vi "Close MeasurementLink Session.vi"(8 "error in":errorcluster, 9 "initialize and close session behavior":T1, 10 "session in":variant, 11 "instrument in":refnum<class "Instrument.lvclass">) -> (0 "error out":errorcluster)   [LabVIEW 2020, in "MeasurementLink niDMM.lvlib" / "Instrument.lvclass"]
uses:
  Instrument.lvclass
  MeasurementLink Measurement Server/Helpers/Error Strings Global Internal.vi
  Instrument.lvclass/Instrument.ctl
  MeasurementLink Instrument/IInstrument/IInstrument.lvclass
  MeasurementLink Instrument/IInstrument/Initialize and Close Session Behavior.ctl
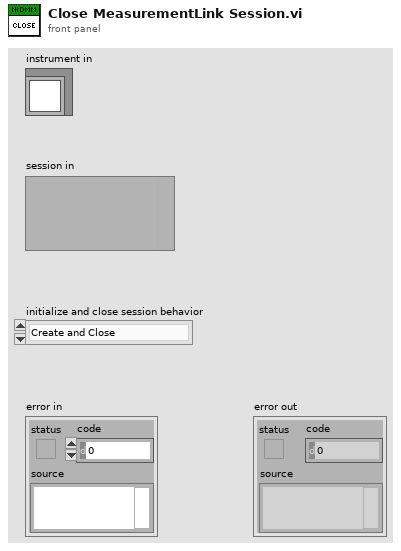
[diagram p1: front panel]
types:
  T1 = typedef "MeasurementLink Instrument.lvlib/IInstrument.lvclass/Initialize and Close Session Behavior.ctl" = enum16{"Create and Close", "Attach and Detach", "Create and Detach", "Attach and Close"}
  T2 = typedef "MeasurementLink Instrument.lvlib/IInstrument.lvclass/Close Session Behavior.ctl" = enum16{"Close Session", "Detach Session"}
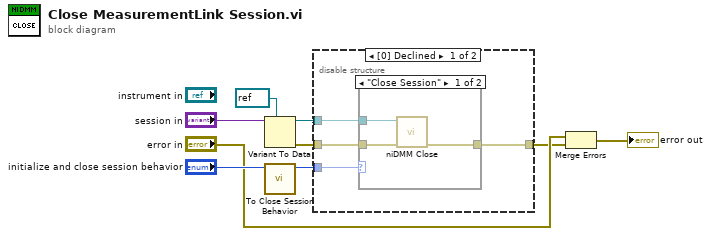
[diagram p0: block diagram]
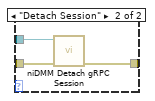
[diagram p2: hidden frame]
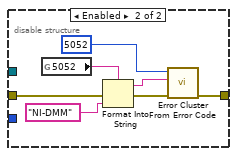
[diagram p3: hidden frame]
diagram:
  n1 = Variant To Data(type=refnum<k15> refnum ("instrument handle"), Variant="session in") -> (data=w6:refnum<k15>, error out=w7:errorcluster)  [unwired: 1 in]
  n2 = call "To Close Session Behavior.vi"("initialize and close session behavior"="initialize and close session behavior") -> ("close session behavior"=w1:T2)  [unwired: 10 in]
  n3 = disable-structure shown="[0] Declined" {
    disable-tunnel: w1 -> [w13 _]
    disable-tunnel: w7 -> [w12 w20]
    disable-tunnel: w6 -> [w11 _]
    disable-tunnel: [w10 w26] -> w3
    frame Disabled {
      n4 = case shown="\"Close Session\"" w13 {
        tunnel: w12 -> [w16 w19]
        tunnel: w11 -> [w15 w17]
        tunnel: [w14 w18] -> w10
        frame "Close Session" {
          n5 = call <instrlib>:"niDMM Close.vi"("error in (no error)"=w16, "instrument handle"=w15) -> ("error out"=w14:errorcluster)  [unwired: 9 in]
        }
        frame "Detach Session" {
          n6 = call <instrlib>:"niDMM Detach gRPC Session.vi"("error in (no error)"=w19, "instrument handle"=w17) -> ("error out"=w18:errorcluster)  [unwired: 9 in]
        }
      }
    }
    frame Enabled {
      n7 = global read "Error Strings Global Internal.vi" "5052"() -> (w24:string)
      n8 = Format Into String(format string=w24, error in=w20, "NI-DMM") -> (resulting string=w21:string, error out=w22:errorcluster)  [unwired: 1 in]
      n9 = call <vilib>:"Error Cluster From Error Code.vi"("error in (no error)"=w22, "error message (\"\")"=w21, "error code (0)"=5052) -> ("error out"=w26:errorcluster)  [unwired: 6 in]
    }
  }
  n10 = Merge Errors("error in", w3) -> (→"error out":errorcluster)
